vi "Get Ingredients.vi"(8 "error in (no error)":errorcluster, 11 "Item in":refnum<class "Item.lvclass">) -> (0 "error out":errorcluster, 2 "Ingredients":T1[](array[typedef]), 3 "Item out":refnum<class "Item.lvclass">)   [LabVIEW 2020, in "Item.lvclass"]
uses:
  Item.lvclass
  Ingredient.ctl
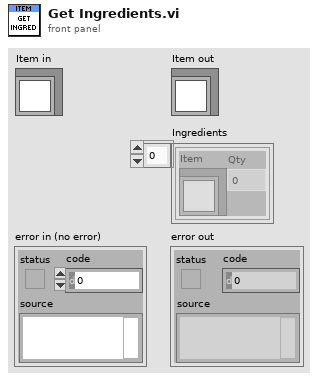
[diagram p1: front panel]
types:
  T1 = typedef "Item.lvclass/Ingredient.ctl" = cluster{"Item":refnum<class "Item.lvclass">, "Qty":dbl}
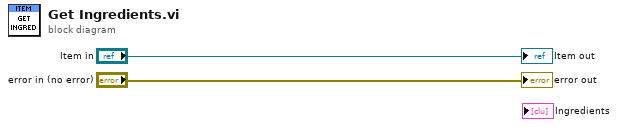
[diagram p0: block diagram]
diagram:
  "error out" <- "error in (no error)"
  "Item out" <- "Item in"
